vi "MeasureTemperatureDiode.vi"() -> (0 "Voltage1":dbl, 1 "Celcius":dbl, 2 "Kelvin":dbl, 3 "Voltage2":dbl)   [LabVIEW 2009]
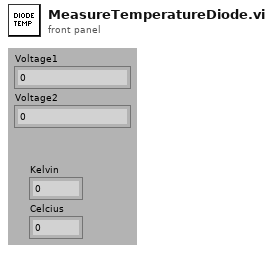
[diagram p1: front panel]
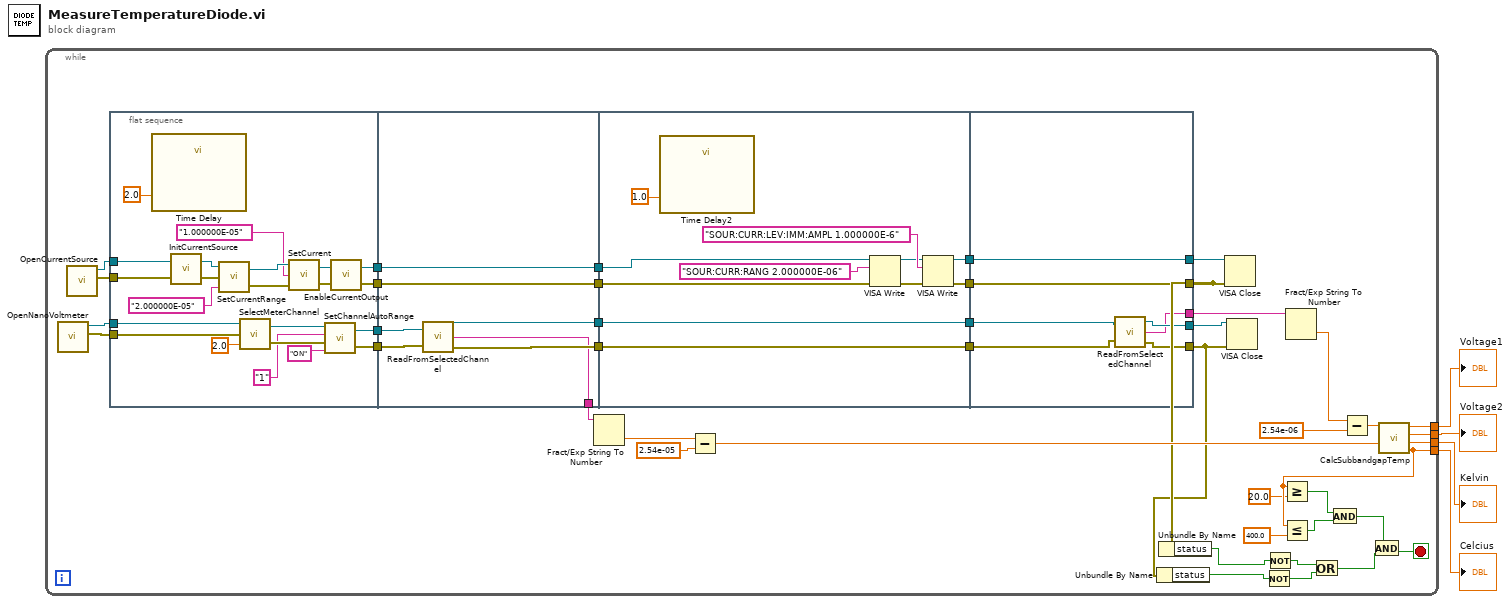
[diagram p0: block diagram]
diagram:
  n1 = while {
    tunnel: [w32] -> w4
    tunnel: [w18] -> w3
    tunnel: [w31] -> w2
    tunnel: [w30] -> w1
    stop <- w5 stop-if-true
    n2 = call "OpenNanoVoltmeter.vi"() -> ("error out"=w23:errorcluster, "reference out"=w22:refnum<visa-resource-name>)  [unwired: 8 in]
    n3 = call "OpenCurrentSource.vi"() -> ("error out"=w20:errorcluster, "reference out"=w21:refnum<visa-resource-name>)  [unwired: 10 in]
    n4 = flat-sequence {
      tunnel: w21 -> [w69]
      tunnel: w20 -> [w68]
      tunnel: [w61] -> w47
      tunnel: [w60] -> w46
      tunnel: [w59] -> w45
      tunnel: [w58] -> w44
      tunnel: w22 -> [w54]
      tunnel: w23 -> [w53]
      tunnel: [w76] -> w43
      tunnel: w47 -> [w76]
      tunnel: [w75] -> w42
      tunnel: w46 -> [w75]
      tunnel: [w74] -> w41
      tunnel: [w73] -> w40
      tunnel: [w72] -> w34
      tunnel: w45 -> [w71]
      tunnel: w44 -> [w70]
      tunnel: w43 -> [w87]
      tunnel: w42 -> [w86]
      tunnel: [w81] -> w39
      tunnel: w41 -> [w81]
      tunnel: [w80] -> w38
      tunnel: w40 -> [w80]
      tunnel: [w79] -> w37
      tunnel: [w78] -> w36
      tunnel: w39 -> [w92]
      tunnel: w38 -> [w91]
      tunnel: w37 -> [w93]
      tunnel: w36 -> [w94]
      tunnel: [w94] -> w19
      tunnel: [w90] -> w13
      tunnel: [w89] -> w35
      tunnel: [w88] -> w33
      tunnel: [w93] -> w14
      frame #0 {
        n5 = call "Time Delay"("Delay Time (s)"=2.0) -> ()  [unwired: 10 in, 1 out]
        n6 = call "InitCurrentSource.vi"("error out 2"=w68, "reference out 2"=w69) -> ("error out"=w67:errorcluster, "reference out"=w66:refnum<visa-resource-name>)
        n7 = call "SetCurrentRange.vi"("string"="2.000000E-05", "error out 2"=w67, "reference out 2"=w66) -> ("error out"=w64:errorcluster, "reference out"=w65:refnum<visa-resource-name>)
        n8 = call "SelectMeterChannel.vi"("ChannelSelection"=2.0, "error out"=w53, "reference out"=w54) -> ("error out 2"=w56:errorcluster, "reference out 2"=w57:refnum<visa-resource-name>)
        n9 = call "SetCurrent.vi"("error out 2"=w64, "string"="1.000000E-05", "reference out 2"=w65) -> ("error out"=w62:errorcluster, "reference out"=w63:refnum<visa-resource-name>)
        n10 = call "SetChannelAutoRange.vi"("On/Off"="ON", "error out 2"=w56, "Channel"="1", "reference out 2"=w57) -> ("error out"=w58:errorcluster, "reference out 3"=w59:refnum<visa-resource-name>)
        n11 = call "EnableCurrentOutput.vi"("error out 2"=w62, "reference out 2"=w63) -> ("error out"=w60:errorcluster, "reference out"=w61:refnum<visa-resource-name>)
      }
      frame #1 {
        n12 = call "ReadFromSelectedChannel.vi"("reference out 3"=w71, "error out"=w70) -> ("reference out 4"=w74:refnum<visa-resource-name>, "read buffer"=w72:string, "error out 2"=w73:errorcluster)
      }
      frame #2 {
        n13 = call "Time Delay2"("Delay Time (s)"=1.0) -> ()  [unwired: 10 in, 1 out]
        n14 = VISA Write(VISA resource name=w87, write buffer="SOUR:CURR:RANG 2.000000E-06", error in (no error)=w86) -> (VISA resource name out=w83:refnum<visa-resource-name>, error out=w82:errorcluster)  [unwired: 1 out]
        n15 = VISA Write(VISA resource name=w83, write buffer="SOUR:CURR:LEV:IMM:AMPL 1.000000E-6", error in (no error)=w82) -> (VISA resource name out=w78:refnum<visa-resource-name>, error out=w79:errorcluster)  [unwired: 1 out]
      }
      frame #3 {
        n16 = call "ReadFromSelectedChannel.vi"("reference out 3"=w92, "error out"=w91) -> ("reference out 4"=w89:refnum<visa-resource-name>, "read buffer"=w88:string, "error out 2"=w90:errorcluster)
      }
    }
    n17 = Fract/Exp String To Number(string=w34) -> (number=w29:dbl)  [unwired: 3 in, 1 out]
    n18 = Subtract(x=w29, y=2.54e-05) -> (x-y=w24:dbl)
    n19 = Unbundle By Name(w13) -> ("status"=w10:bool)
    n20 = Unbundle By Name(w14) -> ("status"=w11:bool)
    n21 = VISA Close(VISA resource name=w19, error in (no error)=w14) -> ()  [unwired: 1 out]
    n22 = VISA Close(VISA resource name=w35, error in (no error)=w13) -> ()  [unwired: 1 out]
    n23 = Not(x=w10) -> (.not. x?=w8:bool)
    n24 = Not(x=w11) -> (.not. x?=w9:bool)
    n25 = Fract/Exp String To Number(string=w33) -> (number=w26:dbl)  [unwired: 3 in, 1 out]
    n26 = Or(x=w9, y=w8) -> (x .or. y?=w6:bool)
    n27 = Subtract(x=w26, y=2.54e-06) -> (x-y=w25:dbl)
    n28 = call "CalcSubbandgapTemp.vi"("Voltage 2"=w25, "Voltage 1"=w24) -> ("Voltage 1"=w31:dbl, "Voltage2"=w30:dbl, "Kelvin"=w32:dbl, "Celcius"=w18:dbl)  [unwired: 1 in]
    n29 = Greater Or Equal?(x=w18, y=20.0) -> (x >= y?=w16:bool)
    n30 = Less Or Equal?(x=w18, y=400.0) -> (x <= y?=w15:bool)
    n31 = And(x=w16, y=w15) -> (x .and. y?=w7:bool)
    n32 = And(x=w7, y=w6) -> (x .and. y?=w5:bool)
  }
  "Kelvin" <- w4
  "Celcius" <- w3
  "Voltage1" <- w2
  "Voltage2" <- w1
